vi "fetch_trajectory.vi"(8 "error in (no error)":errorcluster, 11 "GenericScanHead in":refnum<class "GenericScanHead.lvclass">) -> (0 "error out":errorcluster, 3 "GenericScanHead out":refnum<class "GenericScanHead.lvclass">)   [LabVIEW 2010, in "GenericScanHead.lvclass"]
uses:
  GenericScanHead.lvclass
  Trajectory/GenericTrajectory/GenericTrajectory/GenericTrajectory.lvclass
  class_data.vi
  common/classes/ErrorController/ErrorController/class_data.vi
  common/classes/ErrorController/ErrorController/ErrorController.lvclass
panel:
  out "# elements in queue":i32
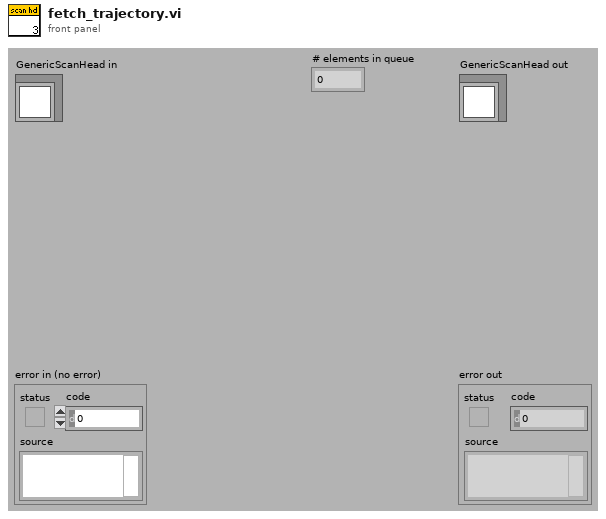
[diagram p1: front panel]
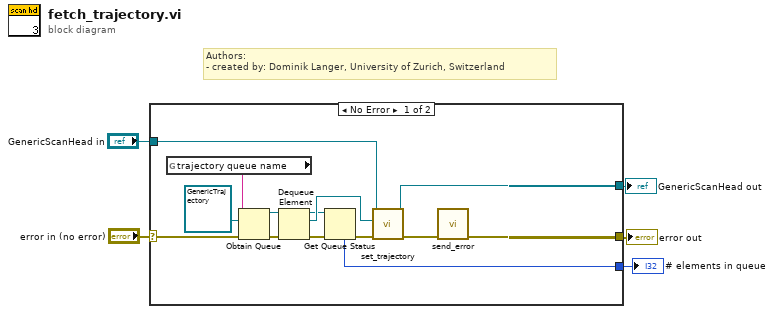
[diagram p0: block diagram]
diagram:
  # "Authors: \n- created by: Dominik Langer, University of Zurich, Switzerland"
  n1 = case shown="No Error" "error in (no error)" {
    selector: "error in (no error)" -> [w18 w21]
    tunnel: [w13 w21] -> w4
    tunnel: [w16 w20] -> w2
    tunnel: "GenericScanHead in" -> [w17 w20]
    tunnel: [w11 _] -> w1
    frame No Error {
      n2 = global read "class_data.vi" "trajectory queue name"() -> (w15:string)
      n3 = Obtain Queue(name (unnamed)=w15, element data type=refnum<class "GenericTrajectory.lvclass"> refnum ("GenericTrajectory.lvclass"), error in (no error)=w18) -> (queue out=w9:refnum<queue>, error out=w10:errorcluster)  [unwired: 2 in, 1 out]
      n4 = Dequeue Element(queue=w9, error in (no error)=w10) -> (queue out=w8:refnum<queue>, element=w12:refnum<class "GenericTrajectory.lvclass">, error out=w7:errorcluster)  [unwired: 2 out]
      n5 = Get Queue Status(queue=w8, error in (no error)=w7) -> (error out=w6:errorcluster, # elements in queue=w11:i32)  [unwired: 1 in, 6 out]
      n6 = call-dynamic "set_trajectory.vi"("error in (no error)"=w6, "trajectory"=w12, "GenericScanHead.lvclass in"=w17) -> ("error out"=w14:errorcluster, "GenericScanHead.lvclass out"=w16:refnum<class "GenericScanHead.lvclass">)  [unwired: 7 out]
      n7 = call "send_error.vi"("error in (no error)"=w14) -> ("error out"=w13:errorcluster)  [unwired: 10 in]
    }
    frame Error {
    }
  }
  "error out" <- w4
  "GenericScanHead out" <- w2
  "# elements in queue" <- w1
